vi "Work Paper No Record2.vi"(8 "error in (no error)":errorcluster, 10 "Main Process Class in":refnum<class "Main Class.lvclass">, 11 "Btn_AutoRun":refnum<vi>) -> ()   [LabVIEW 2019]
uses:
  Main Class.lvclass
  LLB/Commonly VI/Main Glb.vi
  LLB/Commonly VI.lvlib
  <vilib>/NI/Modbus Library/API/Master/Modbus Master.lvclass
panel:
  out "Main Process Class out":refnum<class "Main Class.lvclass">
  in  "Boolean":bool
  out "queue out":refnum<queue>
  out "register values":u16[](array[numeric])
  out "discrete inputs":bool[](array[boolean])
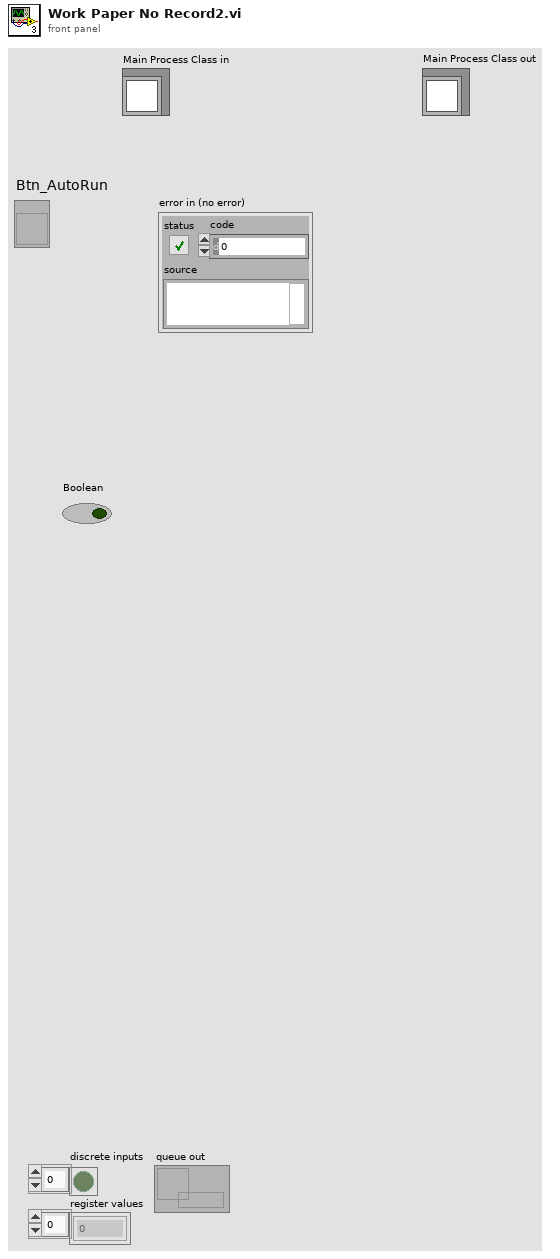
[diagram p1: front panel]
types:
  T1 = cluster{"AutoRunFlg":refnum<vi>, "Action Finish Flg":refnum<vi>, "Remaining Action":refnum<vi>, "Btn_AutoRun":refnum<vi>, "Manual Flg":refnum<vi>, "Sub Process Error":refnum<vi>}
  T2 = cluster{"starting address":u16, "coils to write":bool[]}
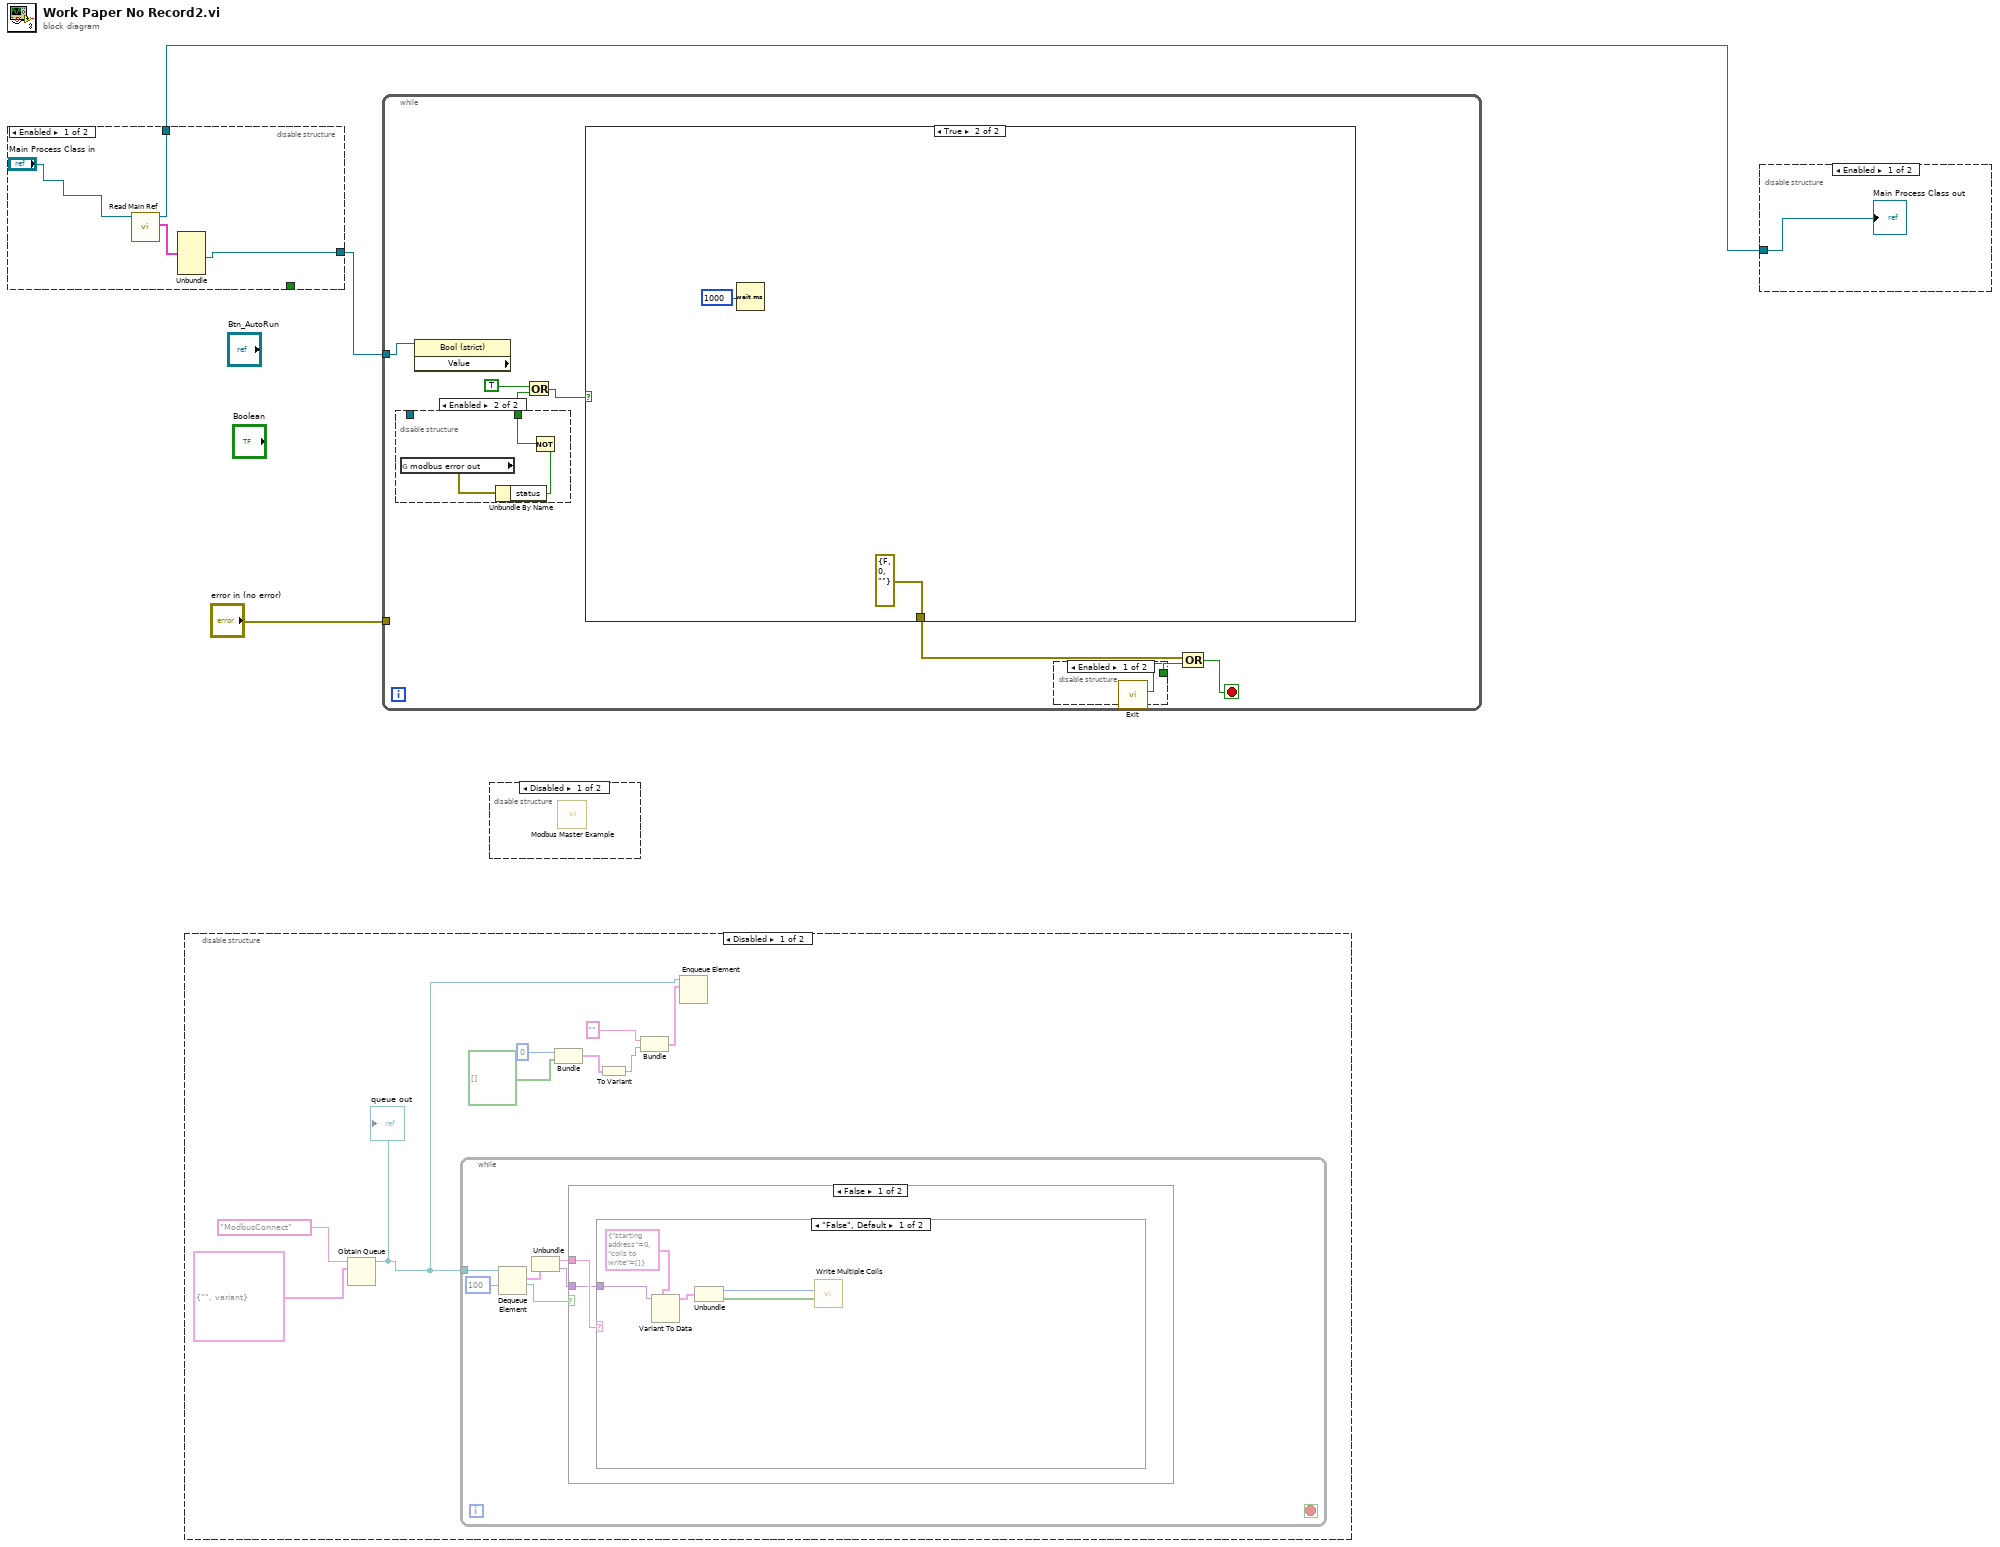
[diagram p0: block diagram]
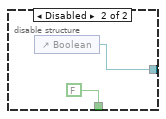
[diagram p4: hidden frame]
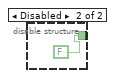
[diagram p5: hidden frame]
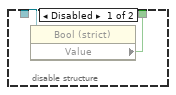
[diagram p6: hidden frame]
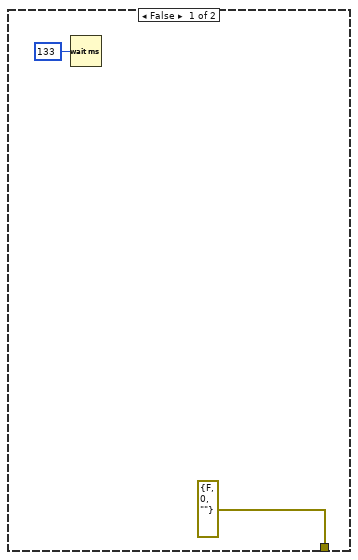
[diagram p7: hidden frame]
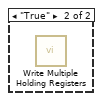
[diagram p8: hidden frame]
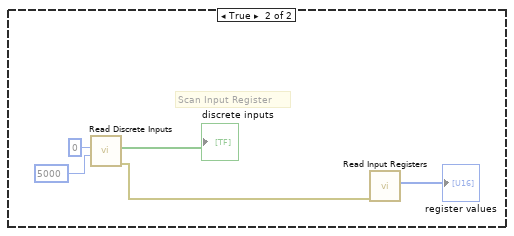
[diagram p9: hidden frame]
diagram:
  n1 = disable-structure shown="Enabled" {
    disable-tunnel: [w6 _] -> w3
    disable-tunnel: [_ FALSE] -> _
    disable-tunnel: [w5 w8] -> w2
    frame Enabled {
      n2 = call-dynamic "Read Main Ref.vi"("Main Process Class in"="Main Process Class in") -> ("Main Ref"=w7:T1, "Main Process Class out"=w6:refnum<class "Main Class.lvclass">)  [unwired: 8 in, 1 out]
      n3 = Unbundle(w7) -> ("Btn_AutoRun"=w5:refnum<vi>)  [unwired: 5 out]
    }
    frame Disabled {
      n4 = control-ref of="Boolean"() -> (w8:refnum<vi>)
    }
  }
  n5 = disable-structure shown="Disabled" {
    frame Disabled {
      n6 = Obtain Queue(name (unnamed)="ModbusConnect", element data type=cluster{string, variant} {"", variant}) -> (queue out=w10:refnum<queue>)  [unwired: 3 in, 2 out]
      "queue out" <- w10
      n7 = while {
        tunnel: w10 -> [w22]
        stop <- _ stop-if-true
        n8 = Dequeue Element(queue=w22, timeout in ms (-1)=100) -> (element=w21:cluster{string, variant}, timed out?=w23:bool)  [unwired: 1 in, 2 out]
        n9 = Unbundle(w21) -> (w20:string, w19:variant)
        n10 = case shown="False" w23 {
          tunnel: w20 -> [w26 _]
          tunnel: w19 -> [w25 _]
          frame False {
            n11 = case shown="\"False\", Default" w26 {
              tunnel: w25 -> [w31 _]
              frame "False", Default {
                n12 = Variant To Data(type=T2 {"starting address"=0, "coils to write"=[]} ("output cluster"), Variant=w31) -> (data=w29:T2)  [unwired: 1 in, 1 out]
                n13 = Unbundle(w29) -> ("starting address"=w28:u16, "coils to write"=w27:bool[])
                n14 = call-dynamic "Write Multiple Coils.vi"("coils to write"=w27, "starting address"=w28) -> ()  [unwired: 8 in, 2 out]
              }
              frame "True" {
                n15 = call-dynamic "Write Multiple Holding Registers.vi"() -> ()  [unwired: 10 in, 2 out]
              }
            }
          }
          frame True {
            # "Scan Input Register"
            n16 = call-dynamic "Read Discrete Inputs.vi"("number of inputs"=u16 5000 ("starting address"), "starting address"=u16 0) -> ("error out"=w33:errorcluster, "discrete inputs"=→"discrete inputs":bool[])  [unwired: 7 in, 1 out]
            n17 = call-dynamic "Read Input Registers.vi"("error in"=w33) -> ("register values"=→"register values":u16[])  [unwired: 8 in, 2 out]
          }
        }
      }
      n18 = Bundle("starting address"=u16 0, "coils to write"=bool[] []) -> (w15:T2)  [unwired: 1 in]
      n19 = To Variant(anything=w15) -> (Variant=w14:variant)
      n20 = Bundle("", "Variant"=w14) -> (w13:cluster{string, "Variant":variant})  [unwired: 1 in]
      n21 = Enqueue Element(queue=w10, element=w13) -> ()  [unwired: 2 in, 3 out]
    }
    frame Enabled {
    }
  }
  n22 = while {
    tunnel: w2 -> [w41]
    tunnel: "error in (no error)" -> [_]
    stop <- w42 stop-if-true
    n23 = disable-structure shown="Enabled" {
      disable-tunnel: _ -> [w47 _]
      disable-tunnel: [w46 w48] -> w38
      frame Disabled {
        n24 = property class="Bool (strict)"(reference=w47) -> ("Value"=w46:bool)  [unwired: 1 in, 2 out]
      }
      frame Enabled {
        n25 = global read "Main Glb.vi" "modbus error out"() -> (w50:errorcluster)
        n26 = Unbundle By Name(w50) -> ("status"=w49:bool)
        n27 = Not(x=w49) -> (.not. x?=w48:bool)
      }
    }
    n28 = property class="Bool (strict)" props=["Value"](reference=w41) -> ()  [unwired: 1 in, 3 out]
    n29 = Or(x=TRUE, y=w38) -> (x .or. y?=w37:bool)
    n30 = case shown="True" w37 {
      tunnel: [errorcluster {"status"=FALSE, "code"=0, "source"=""} ("error out") errorcluster {"status"=FALSE, "code"=0, "source"=""} ("error out")] -> w40
      frame False {
        n31 = Wait (ms)(milliseconds to wait=u32 133) -> ()  [unwired: 1 out]
      }
      frame True {
        n32 = Wait (ms)(milliseconds to wait=1000) -> ()  [unwired: 1 out]
      }
    }
    n33 = disable-structure shown="Enabled" {
      disable-tunnel: [w44 FALSE] -> w43
      frame Enabled {
        n34 = call "Exit.vi"() -> ("ExitOut"=w44:bool)  [unwired: 11 in]
      }
      frame Disabled {
      }
    }
    n35 = Compound Arithmetic op=OR(w40, w43) -> (w42:bool)
  }
  n36 = disable-structure shown="Disabled" {
    frame Disabled {
      n37 = call <vilib>:"Modbus Master Example.vi"() -> ()  [unwired: 12 in]
    }
    frame Enabled {
    }
  }
  n38 = disable-structure shown="Enabled" {
    disable-tunnel: w3 -> [w55 _]
    frame Enabled {
      "Main Process Class out" <- w55
    }
    frame Disabled {
    }
  }
